vi "RTS Open TDMS Get Headers And Groups.vi"(7 "Debug":bool, 8 "error in (no error)":errorcluster, 10 "Operation":T1(ring)=enum."open (read-only)", 11 "file path":path) -> (0 "Error Out":errorcluster, 3 "Refnum out":refnum<k34>)   [LabVIEW 2016]
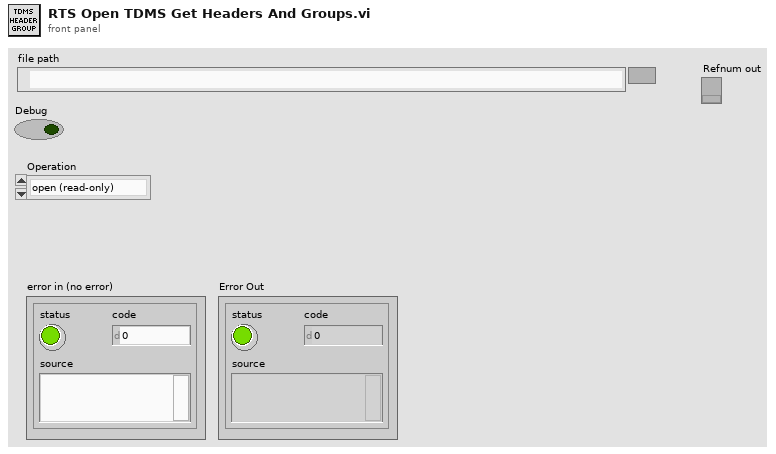
[diagram p1: front panel]
types:
  T1 = enum16{"open", "open or create", "create or replace", "create", "open (read-only)"}
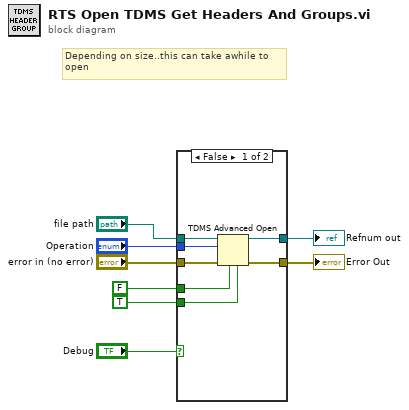
[diagram p0: block diagram]
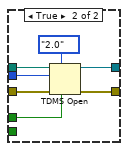
[diagram p2: hidden frame]
diagram:
  # "Depending on size..this can take awhile to\nopen"
  n1 = case shown="False" "Debug" {
    tunnel: "file path" -> [w15 w19]
    tunnel: "error in (no error)" -> [w14 w22]
    tunnel: "Operation" -> [w13 w17]
    tunnel: FALSE ("Disable Buffering? (T)") -> [w12 w16]
    tunnel: [w11 w21] -> w1
    tunnel: [w10 w20] -> w2
    tunnel: TRUE ("enable asynchronous? (T)") -> [w9 _]
    frame False {
      n2 = TDMS Advanced Open(4:w9, 6:w12, 8:w14, 10:w13, 11:w15) -> (0:w11:errorcluster, 3:w10:refnum<k34>)  [unwired: 1 out]
    }
    frame True {
      n3 = TDMS Open(6:w16, 7:enum16{"1.0", "2.0"}."2.0" ("file format version (2.0)"), 8:w22, 10:w17, 11:w19) -> (0:w21:errorcluster, 3:w20:refnum<k34>)  [unwired: 2 in]
    }
  }
  "Refnum out" <- w2
  "Error Out" <- w1
